vi "PA UTSIGNAL.vi"(8 "error in (no error)":errorcluster, 9 "OFF/ON":u16 max=1 step=1, 10 "Step":u16=1 min=1 max=99 step=1, 11 "VISA resource in":refnum<visa-resource-name>) -> (0 "error out":errorcluster, 3 "VISA resource out":refnum<visa-resource-name>)   [LabVIEW 2025]
uses:
  <instrlib>/Chroma 19052/Chroma 19052.lvlib
panel:
  # "Set UT SIGNAL on/off"
  # "0 = OFF\n1 = ON"
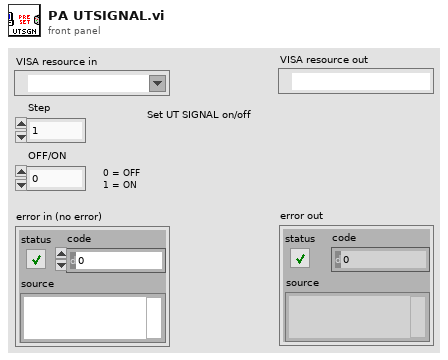
[diagram p1: front panel]
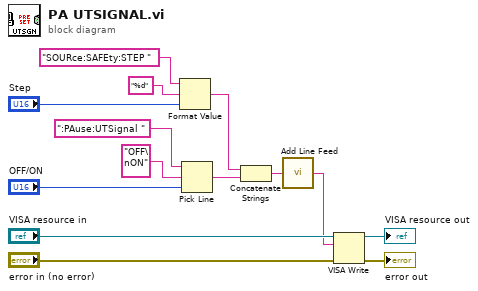
[diagram p0: block diagram]
diagram:
  n1 = Format Value(string ("")="SOURce:SAFEty:STEP ", format string="%d", value (0)="Step") -> (output string=w3:string)
  n2 = Pick Line(string ("")=":PAuse:UTSignal ", multi-line string="OFF\nON", line index="OFF/ON") -> (output string=w4:string)
  n3 = Concatenate Strings(w3, w4) -> (w2:string)
  n4 = call <instrlib>:"Add Line Feed.vi"("Command string"=w2) -> ("Concatenated string"=w1:string)  [unwired: 4 in]
  n5 = VISA Write(VISA resource name="VISA resource in", write buffer=w1, error in (no error)="error in (no error)") -> (VISA resource name out=→"VISA resource out":refnum<visa-resource-name>, error out=→"error out":errorcluster)  [unwired: 1 out]
